vi "Impedance Max and Min vaule.vi"(0 "Horz Time array":dbl[](array[numeric]), 1 "Data In":dbl[](array[numeric]), 3 "Impedance Spec":dbl[](array[numeric])=[110.0, 90.0, 105.0, 95.0], 4 "Cursor List":T1[](array[typedef])) -> (14 "Summary Data":dbl[](array[numeric]), 15 "Summaring Sting":string, 16 "test passed?":bool caption="测试通过？", 17 "Result?":string, 18 "upper Spec":dbl[](array[numeric]), 19 "Lower  Spec":dbl[](array[numeric]))   [LabVIEW 2011]
uses:
  <vilib>/Utility/miscctls.llb/LVPointDoubleTypeDef.ctl
  <vilib>/measure/mamon.llb/Limit Testing Time.vi
  <vilib>/measure/NI_MAPro.lvlib
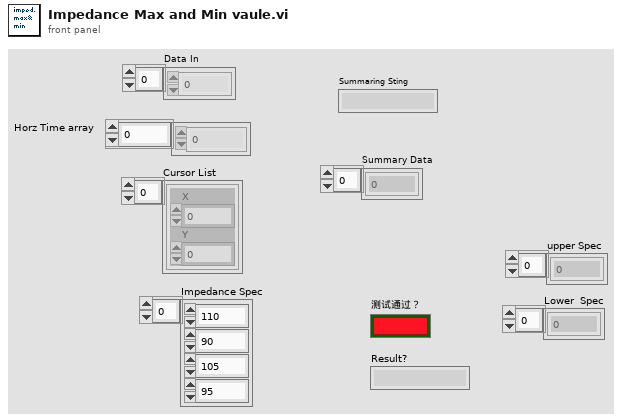
[diagram p1: front panel]
types:
  T1 = typedef "LVPointDoubleTypeDef.ctl" = cluster{"X":dbl, "Y":dbl}
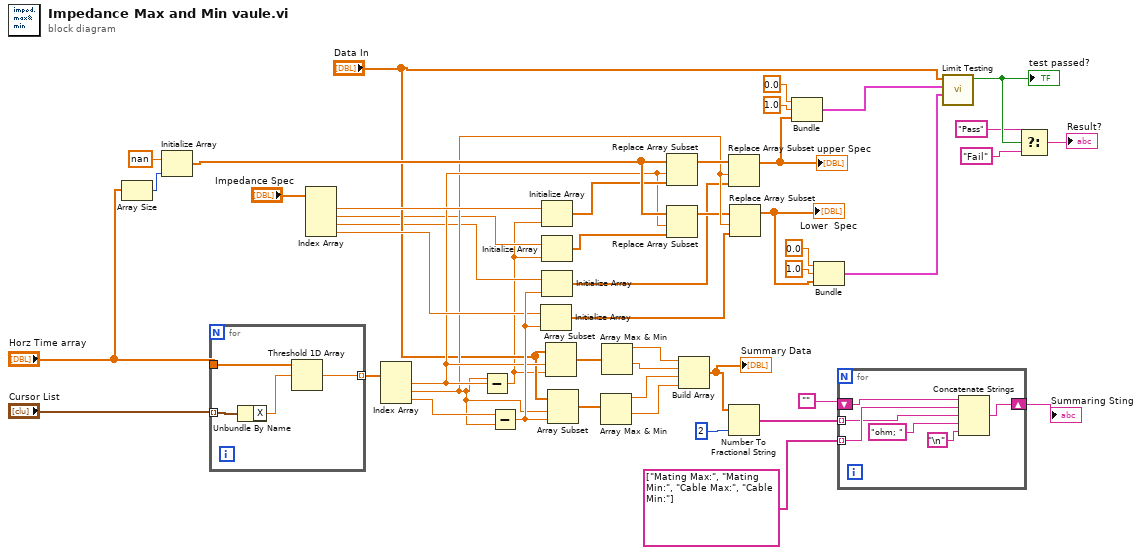
[diagram p0: block diagram]
diagram:
  n1 = Array Size(array="Horz Time array") -> (size(s)=w31:i32)
  n2 = Initialize Array(nan ("元素"), w31) -> (w25:dbl[])
  n3 = for {
    tunnel: "Cursor List" -> [w51] mode=indexing
    tunnel: "Horz Time array" -> [w49]
    tunnel: [w48] -> w46 mode=indexing
    n4 = Unbundle By Name(w51) -> ("X"=w50:dbl)
    n5 = Threshold 1D Array(2:w50, 3:w49) -> (0:w48:dbl)  [unwired: 1 in]
  }
  n6 = Index Array(array="Impedance Spec") -> (element #1=w28:dbl, element #2=w3:dbl, element #3=w2:dbl, element #4=w26:dbl)  [unwired: 4 in]
  n7 = Index Array(array=w46) -> (element #1=w23:dbl, element #2=w21:dbl, element #3=w45:dbl)  [unwired: 3 in]
  n8 = Subtract(x=w21, y=w23) -> (x-y=w1:dbl)
  n9 = Subtract(x=w45, y=w21) -> (x-y=w27:dbl)
  n10 = Initialize Array(w26, w27) -> (w19:dbl[])
  n11 = Initialize Array(w28, w1) -> (w24:dbl[])
  n12 = Initialize Array(w3, w1) -> (w5:dbl[])
  n13 = Initialize Array(w2, w27) -> (w4:dbl[])
  n14 = Array Subset(array="Data In", index=w23, length=w1) -> (w44:dbl[])
  n15 = Array Subset(array="Data In", index=w21, length=w27) -> (w43:dbl[])
  n16 = Array Max & Min(array=w43) -> (max value=w40:dbl, min value=w39:dbl)  [unwired: 2 out]
  n17 = Array Max & Min(array=w44) -> (max value=w42:dbl, min value=w41:dbl)  [unwired: 2 out]
  n18 = Replace Array Subset(array=w25, new element=w24, index=w23) -> (w22:dbl[])
  n19 = Replace Array Subset(array=w25, new element=w5, index=w23) -> (w20:dbl[])
  n20 = Build Array(w42, w41, w40, w39) -> (w38:dbl[])
  "Summary Data" <- w38
  n21 = Replace Array Subset(array=w22, new element=w4, index=w21) -> (w16:dbl[])
  "upper Spec" <- w16
  n22 = Number To Fractional String(number=w38, precision (6)=i16 2 ("精度(6)")) -> (F-format string=w37:string[])  [unwired: 2 in]
  n23 = Replace Array Subset(array=w20, new element=w19, index=w21) -> (w13:dbl[])
  "Lower  Spec" <- w13
  n24 = Bundle("x0"=0.0, "dx"=1.0, w16) -> (w11:cluster{"x0":dbl, "dx":dbl, dbl[]})  [unwired: 1 in]
  n25 = Bundle("x0"=0.0, "dx"=1.0, w13) -> (w10:cluster{"x0":dbl, "dx":dbl, dbl[]})  [unwired: 1 in]
  n26 = for {
    tunnel: w37 -> [w55] mode=indexing
    shift-right: [w53] -> w34
    shift-left: "" -> [w57]
    tunnel: string[] ["Mating Max:", "Mating Min:", "Cable Max:", "Cable Min:"] -> [w56] mode=indexing
    n27 = Concatenate Strings(w57, w56, w55, "ohm; " ("字符串"), "\n") -> (w53:string)
  }
  "Summaring Sting" <- w34
  n28 = call-poly <vilib>:"Limit Testing.vi"("lower limit"=w10, "upper limit"=w11, "signal in"="Data In") -> ("test passed?"=w9:bool)  [unwired: 3 in, 5 out]
  "test passed?" <- w9
  n29 = Select(t="Pass" ("字符串"), s=w9, f="Fail" ("字符串")) -> (s? t:f=→"Result?":string)
